vi "Splash Screen.vi"   [LabVIEW 2019]
uses:
  c4a36dac-c909-414a-aee0-46c6d1a7bcb7.vi
panel:
  # "Jogo da Velha"
  # "®"
types:
  T1 = enum32{"Invalid", "Standard", "Closed", "Hidden", "Minimized", "Maximized"}
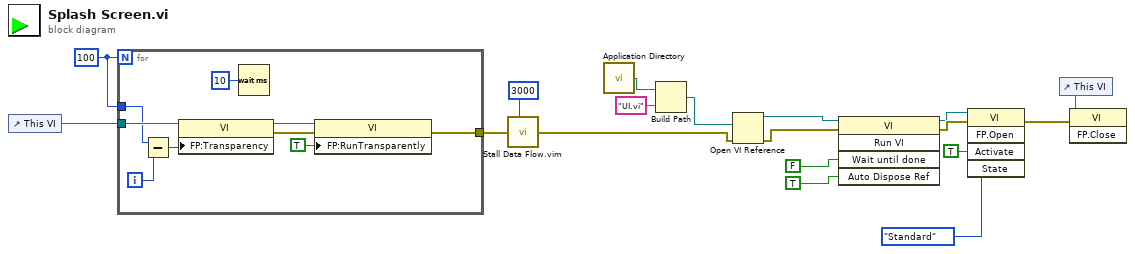
[diagram p0: block diagram]
diagram:
  w17 = 100
  n1 = control-ref of="This VI"() -> (w18:refnum<vi>)
  n2 = for {
    N: w17 -> [_]
    tunnel: w18 -> [w27]
    tunnel: w17 -> [w25]
    tunnel: [w22] -> w8
    i -> [w26]
    n3 = Subtract(x=w25, y=w26) -> (x-y=w19:i32)
    n4 = property on="Property Node" class="VI"(reference=w27, "FP:Transparency"=w19) -> (reference out=w21:refnum<vi>, error out=w24:errorcluster)  [unwired: 1 in]
    n5 = Wait (ms)(milliseconds to wait=u32 10) -> ()  [unwired: 1 out]
    n6 = property class="VI"(reference=w21, error in=w24, "FP:RunTransparently"=TRUE ("Front Panel Window:Run VI Transparently")) -> (error out=w22:errorcluster)  [unwired: 1 out]
  }
  n7 = call "Stall Data Flow.vim"("value in"=w8, "milliseconds to wait"=u32 3000) -> ("value out"=w7:errorcluster)  [unwired: 1 out]
  n8 = call <vilib>:"Application Directory.vi"() -> ("Application Directory"=w16:path)
  n9 = Build Path(base path=w16, name or relative path="UI.vi") -> (appended path=w15:path)
  n10 = Open VI Reference(vi path=w15, error in (no error)=w7) -> (vi reference=w13:refnum<vi>, error out=w10:errorcluster)  [unwired: 4 in]
  n11 = invoke class="VI" method="Run VI"(reference=w13, error in=w10, "Wait until done"=FALSE ("Wait Until Done"), "Auto Dispose Ref"=TRUE ("Auto Dispose Reference")) -> (reference out=w4:refnum<vi>, error out=w9:errorcluster)  [unwired: 1 in, 3 out]
  n12 = invoke class="VI" method="FP.Open"(reference=w4, error in=w9, "Activate"=TRUE ("Activate?"), "State"=T1."Standard") -> (error out=w5:errorcluster)  [unwired: 1 in, 4 out]
  n13 = control-ref of="This VI"() -> (w1:refnum<vi>)
  n14 = invoke class="VI" method="FP.Close"(reference=w1, error in=w5) -> ()  [unwired: 1 in, 3 out]
